vi "Match.vi"(0 "Tolerância X":dbl=300.0, 5 "X Médio":sgl, 7 "Y Médio":sgl, 9 "Tolerância Y":dbl=300.0, 11 "Cluster in":T1) -> (4 "Stop":bool, 8 "Match":bool, 15 "Cluster out":T1)   [LabVIEW 2020]
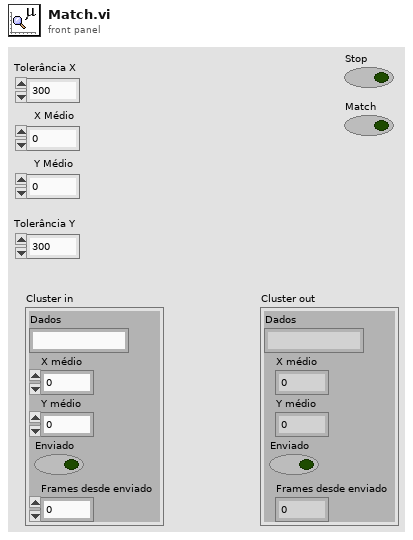
[diagram p1: front panel]
types:
  T1 = cluster{"Dados":string, "X médio":dbl, "Y médio":dbl, "Enviado":bool, "Frames desde enviado":dbl}
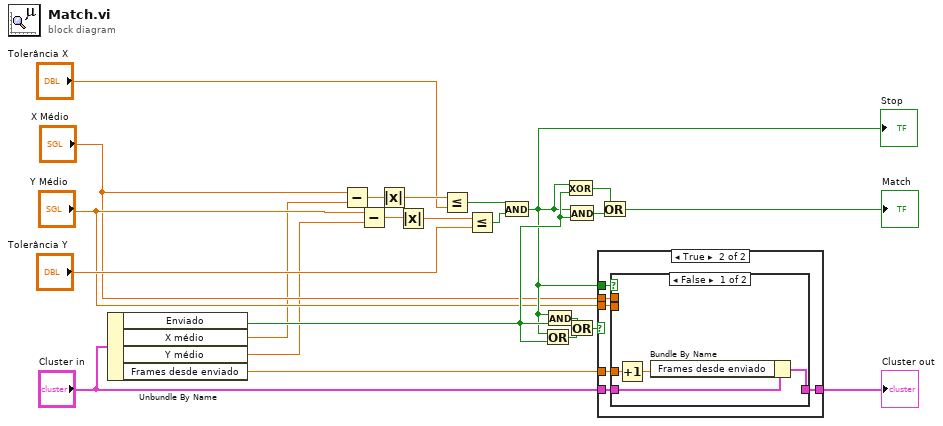
[diagram p0: block diagram]
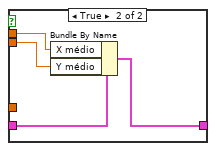
[diagram p3: hidden frame]
diagram:
  n1 = Unbundle By Name("Cluster in") -> ("Enviado"=w23:bool, "X médio"=w1:dbl, "Y médio"=w2:dbl, "Frames desde enviado"=w7:dbl)
  n2 = Subtract(x="X Médio", y=w1) -> (x-y=w12:dbl)
  n3 = Subtract(x="Y Médio", y=w2) -> (x-y=w14:dbl)
  n4 = Absolute Value(x=w12) -> (abs(x)=w13:dbl)
  n5 = Absolute Value(x=w14) -> (abs(x)=w15:dbl)
  n6 = Less Or Equal?(x=w13, y="Tolerância X") -> (x <= y?=w11:bool)
  n7 = Less Or Equal?(x=w15, y="Tolerância Y") -> (x <= y?=w10:bool)
  n8 = And(x=w11, y=w10) -> (x .and. y?=w22:bool)
  "Stop" <- w22
  n9 = Or(x=w22, y=w23) -> (x .or. y?=w21:bool)
  n10 = And(x=w22, y=w23) -> (x .and. y?=w20:bool)
  n11 = Exclusive Or(1:w23, 2:w22) -> (0:w18:bool)
  n12 = And(x=w22, y=w23) -> (x .and. y?=w17:bool)
  n13 = Or(x=w20, y=w21) -> (x .or. y?=w19:bool)
  n14 = case shown="True" w19 {
    tunnel: "Cluster in" -> [w24 w30]
    tunnel: [w24 w29] -> w4
    tunnel: "X Médio" -> [_ w28]
    tunnel: "Y Médio" -> [_ w27]
    tunnel: w7 -> [_ w26]
    tunnel: w22 -> [_ w25]
    frame False {
    }
    frame True {
      n15 = case shown="False" w25 {
        tunnel: w30 -> [w34 w38]
        tunnel: [w33 w37] -> w29
        tunnel: w28 -> [_ w36]
        tunnel: w27 -> [_ w35]
        tunnel: w26 -> [w32 _]
        frame False {
          n16 = Increment(x=w32) -> (x+1=w31:dbl)
          n17 = Bundle By Name(cluster=w34, "Frames desde enviado"=w31) -> (w33:T1)
        }
        frame True {
          n18 = Bundle By Name(cluster=w38, "X médio"=w36, "Y médio"=w35) -> (w37:T1)
        }
      }
    }
  }
  "Cluster out" <- w4
  n19 = Or(x=w18, y=w17) -> (x .or. y?=→"Match":bool)
